vi "HiPOT.vi"(6 "Setting":variant, 8 "error in":errorcluster, 9 "HiPOT Ref":string, 10 "HiPOT Class":string="SIM HiPOT\\SIM HiPOT.lvclass", 11 "Base Path":path=path "C:/GitHub/OOP Template/HAL/Concrete") -> (0 "error out":errorcluster, 3 "Measurements":dbl=0.06305721111028884)   [LabVIEW 2019, in "MAL.lvlib"]
uses:
  MAL.lvlib
  Hardware Abstraction/Harware Abstraction/Analog In/Analog In.lvclass
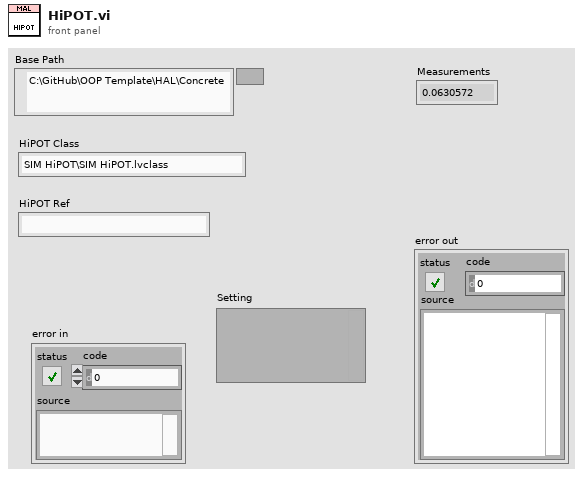
[diagram p1: front panel]
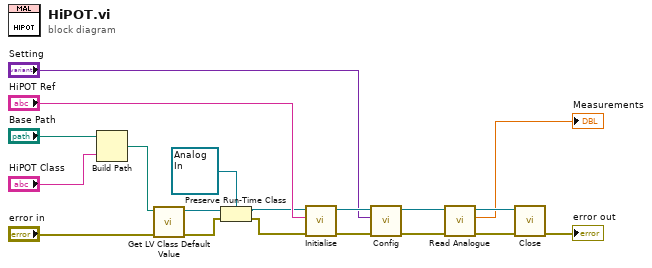
[diagram p0: block diagram]
diagram:
  n1 = Build Path(base path="Base Path", name or relative path="HiPOT Class") -> (appended path=w3:path)
  n2 = call <vilib>:"Get LV Class Default Value.vi"("error in (no error)"="error in", "class path"=w3) -> ("error out"=w17:errorcluster, "object"=w18:refnum<class>)  [unwired: 8 in]
  n3 = Preserve Run-Time Class(object in=w18, error in=w17, 2:refnum<class "Analog In.lvclass"> refnum ("Hardware Abstration.lvlib:Analog In.lvclass")) -> (object out=w15:refnum<class "Analog In.lvclass">, error out=w14:errorcluster)
  n4 = call-dynamic "Initialise.vi"("error in (no error)"=w14, "Instrument Ref"="HiPOT Ref", "Instrument in"=w15) -> ("error out"=w12:errorcluster, "Instrument out"=w11:refnum<class "Analog In.lvclass">)  [unwired: 7 in]
  n5 = call-dynamic "Config.vi"("error in (no error)"=w12, "Setting"="Setting", "Analog In in"=w11) -> ("error out"=w10:errorcluster, "Analog In out"=w9:refnum<class "Analog In.lvclass">)  [unwired: 7 in]
  n6 = call-dynamic "Read Analogue.vi"("error in (no error)"=w10, "PS in"=w9) -> ("error out"=w8:errorcluster, "Measurements"=→"Measurements":dbl, "PS out"=w7:refnum<class "Analog In.lvclass">)  [unwired: 7 in]
  n7 = call-dynamic "Close.vi"("error in (no error)"=w8, "Instrument in"=w7) -> ("error out"=→"error out":errorcluster)  [unwired: 8 in, 1 out]
